vi "Convert directory.vi"(8 "error in (no error)":errorcluster, 9 "directory out":path, 10 "directory in":path, 11 "DAQMH121119OrcaFlash in":refnum<class "DAQOrcaFlash.lvclass">) -> (0 "error out":errorcluster, 3 "DAQMH121119OrcaFlash out":refnum<class "DAQOrcaFlash.lvclass">)   [LabVIEW 2012, in "DAQOrcaFlash.lvclass"]
uses:
  DAQOrcaFlash.lvclass
  DAQOrcaFlash.lvclass/DAQOrcaFlash.ctl
  <vilib>/Zen Informatics/Zen Image/ImageCollection/ImageCollection.lvclass
  <vilib>/Zen Informatics/Zen Image/Image/Image.lvclass
  <vilib>/Zen Informatics/Zen Image/Image/storage_mode.ctl
  <vilib>/Zen Informatics/Zen Image/ImageCollection/storage_mode_enum.ctl
  <vilib>/Zen Informatics/Zen Image/ImageCollection/add_mode_enum.ctl
panel:
  out "Files written to":path
  out "filename":string
  out "progress bar":sgl(slide) scale=0.0..1.0
  out "x+y":sgl
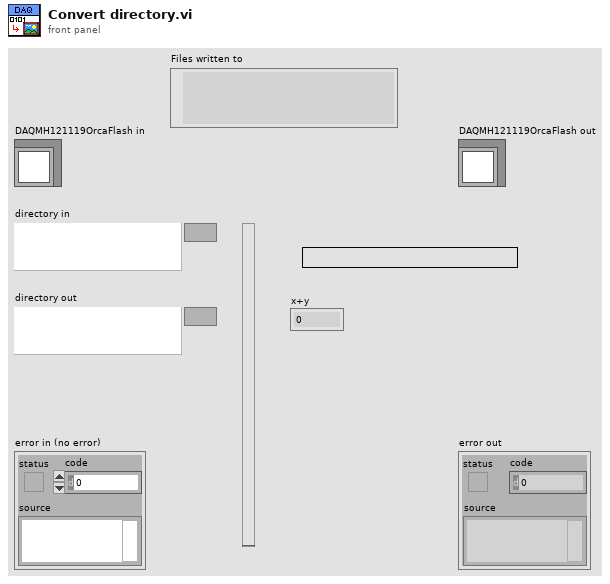
[diagram p1: front panel]
types:
  T1 = typedef "ImageCollection.lvclass/storage_mode_enum.ctl" = enum16{"RAM", "single files", "multipage TIFF (read-only)"}
  T2 = typedef "ImageCollection.lvclass/add_mode_enum.ctl" = enum16{"reference", "copy"}
  T3 = typedef "Image.lvclass/storage_mode.ctl" = enum16{"RAM", "disk"}
  T4 = typedef "Image Type" = u32
  T5 = typedef "IMAQ Image.ctl" = refnum<image>
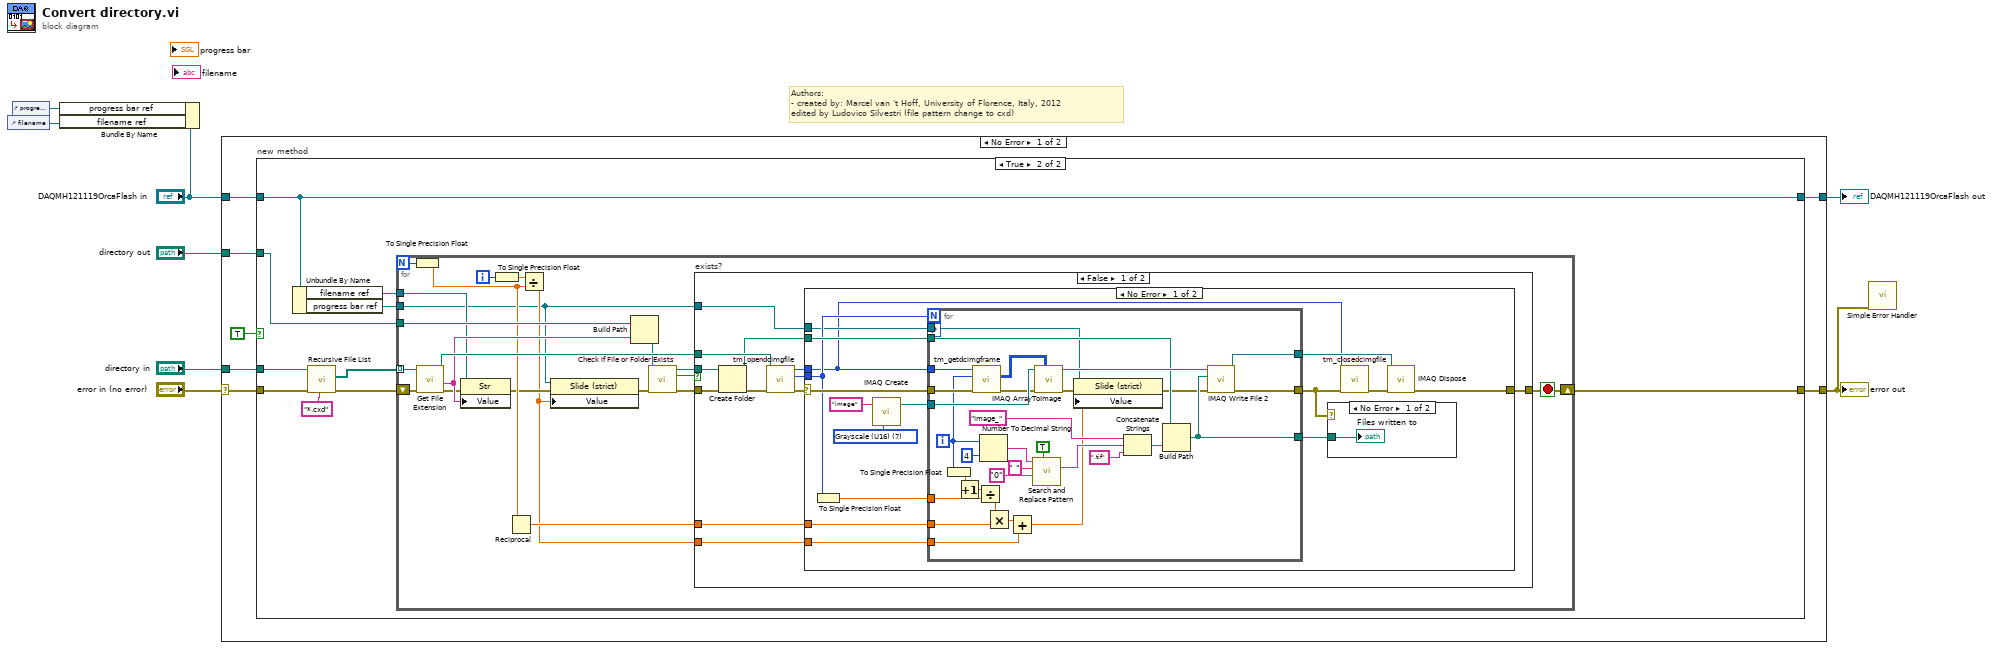
[diagram p0: block diagram]
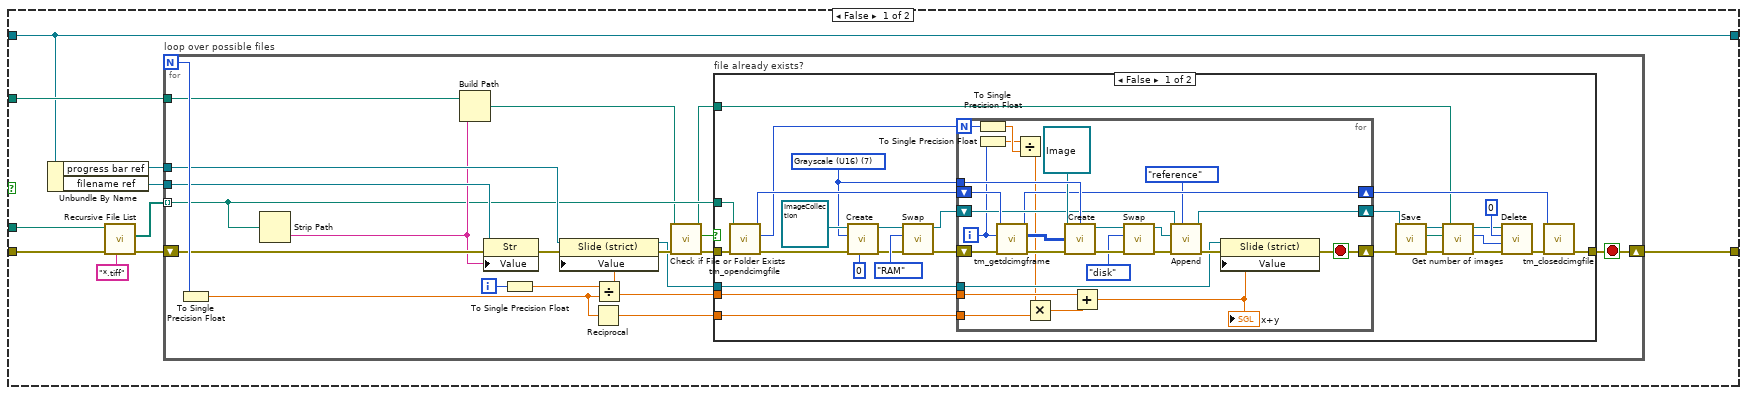
[diagram p2: hidden frame]
diagram:
  # "Authors: \n- created by: Marcel van 't Hoff, University of Florence, Italy, 2012\nedited by Ludovico Silvestri (file pattern change to cxd)"
  n1 = control-ref of="filename"() -> (w4:refnum<vi>)
  n2 = control-ref of="progress bar"() -> (w5:refnum<vi>)
  n3 = Bundle By Name(cluster="DAQMH121119OrcaFlash in", "progress bar ref"=w5, "filename ref"=w4) -> ()  [unwired: 1 out]
  n4 = case shown="No Error" "error in (no error)" {
    selector: "error in (no error)" -> [w14 w196]
    tunnel: [w11 w196] -> w2
    tunnel: [w10 w195] -> w8
    tunnel: "DAQMH121119OrcaFlash in" -> [w13 w195]
    tunnel: "directory in" -> [w15 _]
    tunnel: "directory out" -> [w12 _]
    frame No Error {
      n5 = case "new method" shown="True" TRUE {
        tunnel: w15 -> [w25 w109]
        tunnel: w14 -> [w24 w107]
        tunnel: w13 -> [w16 w104]
        tunnel: w12 -> [w18 w105]
        tunnel: [w17 w111] -> w11
        tunnel: [w16 w104] -> w10
        frame False {
          n6 = Unbundle By Name(w16) -> ("progress bar ref"=w20:refnum<vi>, "filename ref"=w19:refnum<vi>)
          n7 = call <vilib>:"Recursive File List.vi"("pattern"="*.tiff", "error in (no error)"=w24, "Folder Path"=w25) -> ("error out"=w21:errorcluster, "All Files in Dir"=w22:path[])  [unwired: 4 in, 3 out]
          n8 = for "loop over possible files" {
            N -> [w45]
            tunnel: w22 -> [w35] mode=indexing
            shift-right: [w36] -> w17
            shift-left: w21 -> [w42]
            tunnel: w20 -> [w43]
            tunnel: w19 -> [w41]
            tunnel: w18 -> [w40]
            i -> [w44]
            stop <- w36 stop-if-true
            n9 = To Single Precision Float(number=w45) -> (single precision float=w27:sgl)
            n10 = Strip Path(path=w35) -> (name=w39:string)  [unwired: 1 out]
            n11 = Build Path(base path=w40, name or relative path=w39) -> (appended path=w34:path)
            n12 = property class="Str"(reference=w41, error in=w42, "Value"=w39) -> (error out=w37:errorcluster)  [unwired: 1 out]
            n13 = To Single Precision Float(number=w44) -> (single precision float=w38:sgl)
            n14 = Reciprocal(x=w27) -> (1/x=w26:sgl)
            n15 = Divide(x=w38, y=w27) -> (x/y=w29:sgl)
            n16 = property class="Slide (strict)"(reference=w43, error in=w37, "Value"=w29) -> (reference out=w28:refnum<vi>, error out=w32:errorcluster)
            n17 = call <vilib>:"Check if File or Folder Exists.vi"("error in (no error)"=w32, "path"=w34) -> ("error out"=w31:errorcluster, "file or folder exists?"=w30:bool, "dup path"=w33:path)  [unwired: 7 in]
            n18 = case "file already exists?" shown="False" w30 {
              tunnel: [w57 w101] -> w36
              tunnel: w35 -> [w56 _]
              tunnel: w33 -> [w55 _]
              tunnel: w31 -> [w54 w101]
              tunnel: w29 -> [w53 _]
              tunnel: w28 -> [w52 _]
              tunnel: w26 -> [w51 _]
              frame False {
                w70 = T4 7 items=["Grayscale (U8)", "Grayscale (I16)", "Grayscale (SGL)", "Complex (CSG)", "RGB (U32)", "HSL (U32)", "RGB (U64)", "Grayscale (U16)"] ("Image Type")
                n19 = call <userlib>:"tm_opendcimgfile.vi"("error in (no error)"=w54, "Path"=w56) -> ("error out"=w72:errorcluster, "Total Frames"=w60:i32, "File Handle"=w71:u32)  [unwired: 7 in]
                n20 = call-dynamic "Create.vi"("size"=0, "error in (no error)"=w72, "Image Type"=w70, "ImageCollection in"=refnum<class "ImageCollection.lvclass"> refnum) -> ("error out"=w47:errorcluster, "ImageCollection out"=w50:refnum<class "ImageCollection.lvclass">)  [unwired: 6 in]
                n21 = call-dynamic "Swap.vi"("error in (no error)"=w47, "target storage mode"=storage_mode_enum."RAM" ("type"), "ImageCollection in"=w50) -> ("error out"=w46:errorcluster, "ImageCollection out"=w49:refnum<class "ImageCollection.lvclass">)  [unwired: 6 in, 1 out]
                n22 = for {
                  N: w60 -> [w86]
                  shift-right: [w80] -> w68
                  shift-left: w46 -> [w99]
                  tunnel: w70 -> [w96]
                  shift-right: [w93] -> w67
                  shift-left: w49 -> [w94]
                  shift-right: [w92] -> w58
                  shift-left: w71 -> [w100]
                  tunnel: w53 -> [w82]
                  tunnel: w52 -> [w78]
                  tunnel: w51 -> [w77]
                  i -> [w83]
                  stop <- w80 stop-if-true
                  n23 = To Single Precision Float(number=w86) -> (single precision float=w85:sgl)
                  n24 = To Single Precision Float(number=w83) -> (single precision float=w84:sgl)
                  n25 = call <userlib>:"tm_getdcimgframe.vi"("error in (no error)"=w99, "Frame Index"=w83, "File Handle in"=w100) -> ("error out"=w97:errorcluster, "Data"=w98:u16[][], "File Handle out"=w92:u32)  [unwired: 5 in, 1 out]
                  n26 = Divide(x=w84, y=w85) -> (x/y=w75:sgl)
                  n27 = Multiply(x=w75, y=w77) -> (x*y=w76:sgl)
                  n28 = call-dynamic "Create.vi"("Image in"=refnum<class "Image.lvclass"> refnum, "Image Type"=w96, "Image Pixels (U16)"=w98, "error in (no error)"=w97) -> ("Image out"=w91:refnum<class "Image.lvclass">, "error out"=w89:errorcluster)  [unwired: 10 in]
                  n29 = Add(x=w82, y=w76) -> (x+y=w79:sgl)
                  "x+y" <- w79
                  n30 = call-dynamic "Swap.vi"("error in (no error)"=w89, "storage type target"=storage_mode."disk" ("storage type"), "Image in"=w91) -> ("error out"=w88:errorcluster, "Image out"=w90:refnum<class "Image.lvclass">)  [unwired: 6 in, 1 out]
                  n31 = call-dynamic "Append.vi"("add mode (copy)"=add_mode_enum."reference", "error in (no error)"=w88, "Image.lvclass"=w90, "ImageCollection in"=w94) -> ("error out"=w81:errorcluster, "ImageCollection out"=w93:refnum<class "ImageCollection.lvclass">)  [unwired: 5 in, 1 out]
                  n32 = property class="Slide (strict)"(reference=w78, error in=w81, "Value"=w79) -> (error out=w80:errorcluster)  [unwired: 1 out]
                }
                n33 = call-dynamic "Save.vi"("error in (no error)"=w68, "path"=w55, "ImageCollection in"=w67) -> ("error out"=w63:errorcluster, "ImageCollection out"=w65:refnum<class "ImageCollection.lvclass">)  [unwired: 7 in]
                n34 = call-dynamic "Get number of images.vi"("error in (no error)"=w63, "ImageCollection in"=w65) -> ("error out"=w62:errorcluster, "size"=w61:i32, "ImageCollection out"=w64:refnum<class "ImageCollection.lvclass">)  [unwired: 7 in]
                n35 = call-dynamic "Delete.vi"("error in (no error)"=w62, "range"=w61, "start index"=0, "ImageCollection in"=w64) -> ("error out"=w59:errorcluster)  [unwired: 6 in, 1 out]
                n36 = call <userlib>:"tm_closedcimgfile.vi"("error in (no error)"=w59, "File Handle"=w58) -> ("error out"=w57:errorcluster)  [unwired: 9 in]
              }
              frame True {
              }
            }
          }
        }
        frame True {
          n37 = Unbundle By Name(w104) -> ("filename ref"=w103:refnum<vi>, "progress bar ref"=w102:refnum<vi>)
          n38 = call <vilib>:"Recursive File List.vi"("pattern"="*.cxd", "error in (no error)"=w107, "Folder Path"=w109) -> ("error out"=w106:errorcluster, "All Files in Dir"=w108:path[])  [unwired: 4 in, 3 out]
          n39 = for {
            N -> [w121]
            tunnel: w108 -> [w130] mode=indexing
            shift-right: [w125] -> w111
            shift-left: w106 -> [w131]
            tunnel: w105 -> [w132]
            tunnel: w103 -> [w122]
            tunnel: w102 -> [w114]
            i -> [w120]
            stop <- w125 stop-if-true
            n40 = To Single Precision Float(number=w121) -> (single precision float=w118:sgl)
            n41 = call <vilib>:"Get File Extension.vi"("error in (no error)"=w131, "file"=w130) -> ("error out"=w123:errorcluster, "filename without extension"=w124:string, "dup file"=w129:path)  [unwired: 6 in, 1 out]
            n42 = property class="Str"(reference=w122, error in=w123, "Value"=w124) -> (error out=w117:errorcluster)  [unwired: 1 out]
            n43 = To Single Precision Float(number=w120) -> (single precision float=w119:sgl)
            n44 = Reciprocal(x=w118) -> (1/x=w116:sgl)
            n45 = Divide(x=w119, y=w118) -> (x/y=w115:sgl)
            n46 = property class="Slide (strict)"(reference=w114, error in=w117, "Value"=w115) -> (error out=w112:errorcluster)  [unwired: 1 out]
            n47 = Build Path(base path=w132, name or relative path=w124) -> (appended path=w113:path)
            n48 = call <vilib>:"Check if File or Folder Exists.vi"("error in (no error)"=w112, "path"=w113) -> ("error out"=w127:errorcluster, "file or folder exists?"=w126:bool, "dup path"=w128:path)  [unwired: 7 in]
            n49 = case "exists?" shown="False" w126 {
              tunnel: [w141 w194] -> w125
              tunnel: w129 -> [w140 _]
              tunnel: w128 -> [w136 _]
              tunnel: w127 -> [w134 w194]
              tunnel: w116 -> [w139 _]
              tunnel: w115 -> [w138 _]
              tunnel: w114 -> [w137 _]
              frame False {
                n50 = Create Folder(path (use dialog)=w136, error in=w134) -> (created path=w135:path, error out=w133:errorcluster)  [unwired: 1 in, 1 out]
                n51 = call <userlib>:"tm_opendcimgfile.vi"("error in (no error)"=w133, "Path"=w140) -> ("error out"=w142:errorcluster, "Total Frames"=w144:i32, "File Handle"=w143:u32)  [unwired: 7 in]
                n52 = case shown="No Error" w142 {
                  selector: w142 -> [w160 w193]
                  tunnel: w143 -> [w145 _]
                  tunnel: [w153 w193] -> w141
                  tunnel: w144 -> [w150 _]
                  tunnel: w135 -> [w155 _]
                  tunnel: w139 -> [w148 _]
                  tunnel: w138 -> [w147 _]
                  tunnel: w137 -> [w146 _]
                  frame No Error {
                    w158 = T4 7 items=["Grayscale (U8)", "Grayscale (I16)", "Grayscale (SGL)", "Complex (CSG)", "RGB (U32)", "HSL (U32)", "RGB (U64)", "Grayscale (U16)"] ("Image Type")
                    n53 = To Single Precision Float(number=w150) -> (single precision float=w149:sgl)
                    n54 = call "IMAQ Create"("Image Name"="image", "Image Type"=w158) -> ("New Image"=w157:T5)  [unwired: 3 in, 1 out]
                    n55 = for {
                      N: w150 -> [_]
                      tunnel: w157 -> [w190]
                      tunnel: w155 -> [w176]
                      tunnel: [w175] -> w152
                      tunnel: [w174] -> w151
                      tunnel: w149 -> [w173]
                      tunnel: w148 -> [w170]
                      tunnel: w147 -> [w167]
                      tunnel: w146 -> [w163]
                      tunnel: w160 -> [w191]
                      tunnel: [w177] -> w156
                      tunnel: w145 -> [w192]
                      workers-P: _ -> [_]
                      i -> [w172]
                      n56 = To Single Precision Float(number=w172) -> (single precision float=w171:sgl)
                      n57 = Increment(x=w171) -> (x+1=w162:sgl)
                      n58 = call <userlib>:"tm_getdcimgframe.vi"("error in (no error)"=w191, "Frame Index"=w172, "File Handle in"=w192) -> ("error out"=w188:errorcluster, "Data"=w178:u16[][])  [unwired: 5 in, 2 out]
                      n59 = Divide(x=w162, y=w173) -> (x/y=w169:sgl)
                      n60 = Number To Decimal String(number=w172, width (-)=i16 4) -> (decimal integer string=w185:string)
                      n61 = Multiply(x=w169, y=w170) -> (x*y=w168:sgl)
                      n62 = Add(x=w168, y=w167) -> (x+y=w166:sgl)
                      n63 = call <vilib>:"Search and Replace Pattern.vi"("string"=w185, "regular expression (\"\")"=" " ("regular expression (\"\")"), "replace string (\"\")"="0" ("replace string (\"\")"), "replace all? (F)"=TRUE) -> ("result string"=w181:string)  [unwired: 1 in, 1 out]
                      n64 = call "IMAQ ArrayToImage"("Image Pixels (U16)"=w178, "error in (no error)"=w188, "Image"=w190) -> ("error out"=w165:errorcluster, "Image Out"=w189:T5)  [unwired: 7 in]
                      n65 = property class="Slide (strict)"(reference=w163, error in=w165, "Value"=w166) -> (error out=w164:errorcluster)  [unwired: 1 out]
                      n66 = Concatenate Strings("image_", w181, ".tif" ("regular expression (\"\")")) -> (w180:string)
                      n67 = Build Path(base path=w176, name or relative path=w180) -> (appended path=w174:path)
                      n68 = call-poly "IMAQ Write File 2"("error in (no error)"=w164, "File Path"=w174, "Image"=w189) -> ("error out"=w177:errorcluster, "Image Out (duplicate)"=w175:T5)  [unwired: 7 in]
                    }
                    n69 = case shown="No Error" w156 {
                      tunnel: w151 -> [w161 _]
                      frame No Error {
                        "Files written to" <- w161
                      }
                      frame Error {
                      }
                    }
                    n70 = call <userlib>:"tm_closedcimgfile.vi"("error in (no error)"=w156, "File Handle"=w145) -> ("error out"=w154:errorcluster)  [unwired: 9 in]
                    n71 = call "IMAQ Dispose"("Image"=w152, "error in (no error)"=w154) -> ("error out"=w153:errorcluster)  [unwired: 4 in]
                  }
                  frame Error {
                  }
                }
              }
              frame True {
              }
            }
          }
        }
      }
    }
    frame Error {
    }
  }
  "error out" <- w2
  "DAQMH121119OrcaFlash out" <- w8
  n72 = call <vilib>:"Simple Error Handler.vi"("error in (no error)"=w2) -> ()  [unwired: 4 in, 5 out]
